vi "Img Update w Point.vi"(8 "error in (no error)":errorcluster, 11 "LF2R IDE in":refnum<class "LF2R IDE.lvclass">) -> (0 "error out":errorcluster, 3 "LF2R IDE out":refnum<class "LF2R IDE.lvclass">)   [LabVIEW 2018, in "LF2R IDE.lvlib" / "LF2R IDE.lvclass"]
uses:
  LF2R IDE.lvclass
  LF2R IDE.lvclass/LF2R IDE.ctl
  Image/Image Process.lvclass
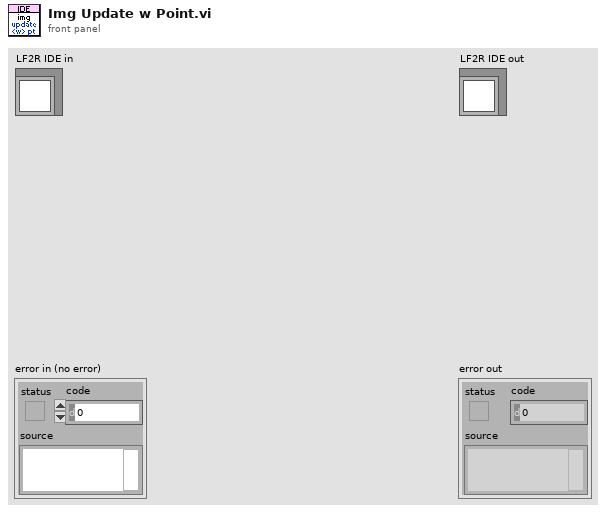
[diagram p1: front panel]
types:
  T1 = typedef "IMAQ Image.ctl" = refnum<image>
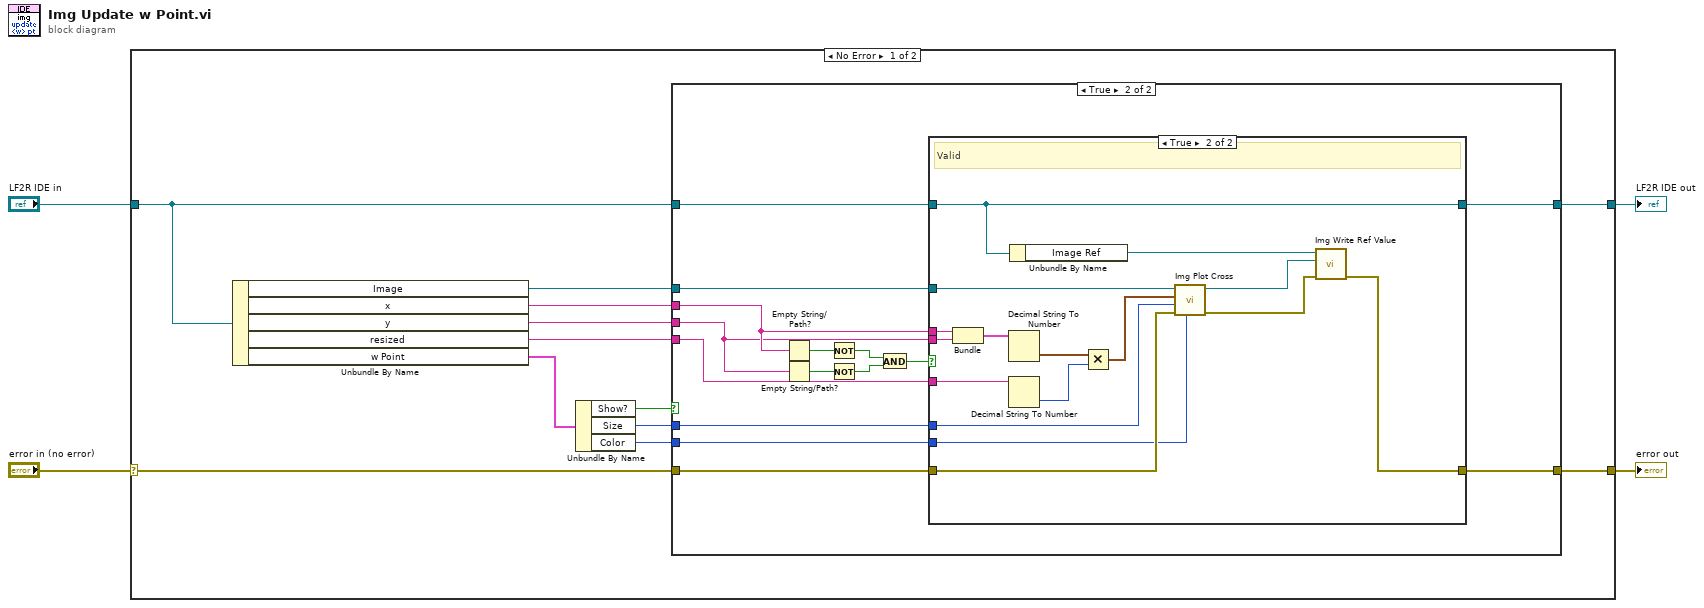
[diagram p0: block diagram]
diagram:
  n1 = case shown="No Error" "error in (no error)" {
    selector: "error in (no error)" -> [w12 w53]
    tunnel: [w15 w53] -> w3
    tunnel: [w9 w52] -> w1
    tunnel: "LF2R IDE in" -> [w16 w52]
    frame No Error {
      n2 = Unbundle By Name(w16) -> ("Image"=w13:T1, "x"=w11:string, "y"=w10:string, "resized"=w14:string, "w Point"=w8:cluster{"Size":i32, "Color":u32, "Show?":bool})
      n3 = Unbundle By Name(w8) -> ("Show?"=w7:bool, "Size"=w6:i32, "Color"=w5:u32)
      n4 = case shown="True" w7 {
        tunnel: w16 -> [w18 w33]
        tunnel: [w17 w32] -> w15
        tunnel: w14 -> [_ w31]
        tunnel: w13 -> [_ w30]
        tunnel: w12 -> [w17 w29]
        tunnel: w11 -> [_ w28]
        tunnel: w10 -> [_ w27]
        tunnel: [w18 w21] -> w9
        tunnel: w6 -> [_ w20]
        tunnel: w5 -> [_ w19]
        frame False {
        }
        frame True {
          n5 = Empty String/Path?(string/path=w28) -> (empty?=w26:bool)
          n6 = Empty String/Path?(string/path=w27) -> (empty?=w25:bool)
          n7 = Not(x=w26) -> (.not. x?=w24:bool)
          n8 = Not(x=w25) -> (.not. x?=w23:bool)
          n9 = And(x=w24, y=w23) -> (x .and. y?=w22:bool)
          n10 = case shown="True" w22 {
            tunnel: w33 -> [w35 w38]
            tunnel: [w34 w50] -> w32
            tunnel: w31 -> [_ w49]
            tunnel: w30 -> [_ w46]
            tunnel: w29 -> [w34 w44]
            tunnel: w28 -> [_ w41]
            tunnel: w27 -> [_ w40]
            tunnel: [w35 w38] -> w21
            tunnel: w20 -> [_ w37]
            tunnel: w19 -> [_ w36]
            frame False {
              # "Invalid"
            }
            frame True {
              # "Valid"
              n11 = Bundle("x"=w41, "y"=w40) -> (w39:cluster{"x":string, "y":string})  [unwired: 1 in]
              n12 = Decimal String To Number(string=w39) -> (number=w48:cluster{"x":i32, "y":i32})  [unwired: 2 in, 1 out]
              n13 = Decimal String To Number(string=w49) -> (number=w47:i32)  [unwired: 2 in, 1 out]
              n14 = Unbundle By Name(w38) -> ("Image Ref"=w51:refnum<vi>)
              n15 = Multiply(x=w48, y=w47) -> (x*y=w45:cluster{"x":i32, "y":i32})
              n16 = call "Img Plot Cross.vi"("Color"=w36, "error in (no error)"=w44, "size"=w37, "position"=w45, "Image In"=w46) -> ("error out"=w43:errorcluster, "Image Out"=w42:T1)  [unwired: 5 in]
              n17 = call "Img Write Ref Value.vi"("error in (no error)"=w43, "Image"=w42, "Image Ref"=w51) -> ("error out"=w50:errorcluster)  [unwired: 8 in]
            }
          }
        }
      }
    }
    frame Error {
    }
  }
  "error out" <- w3
  "LF2R IDE out" <- w1
